vi "From Base Packet.vi"(8 "error in (no error)":errorcluster, 11 "Base Packet":refnum<class "Packet.lvclass">) -> (0 "error out":errorcluster, 3 "Operator out":refnum<class "Operator.lvclass">)   [LabVIEW 2020, in "Operator.lvclass"]
uses:
  Operator.lvclass
  Operator.lvclass/Operator.ctl
  Packet/Packet.lvclass
  C:/dev/IlluminatedG/AdventOfCode/2021/source/Day 16/Part 1/Packet/Packet.lvclass
  C:/dev/IlluminatedG/AdventOfCode/2021/source/Day 16/Part 1/Operator/Operator.lvclass
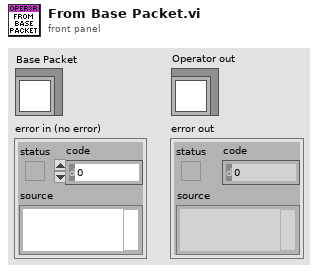
[diagram p1: front panel]
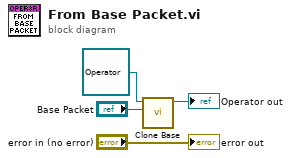
[diagram p0: block diagram]
diagram:
  n1 = call "Clone Base.vi"("From"="Base Packet", "Packet in"=refnum<class "Operator.lvclass"> refnum ("Operator.lvclass")) -> ("Packet out"=→"Operator out":refnum<class "Operator.lvclass">)  [unwired: 8 in, 1 out]
  "error out" <- "error in (no error)"
